vi "manual slider.vi"() -> ()   [LabVIEW 2020]
panel:
  out "Boolean 2":bool
  in  "Boolean":bool
  in  "stop":bool
  in  "VISA resource name":refnum<visa-resource-name>
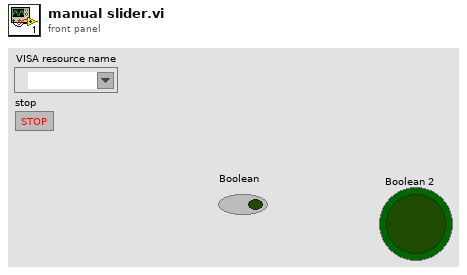
[diagram p1: front panel]
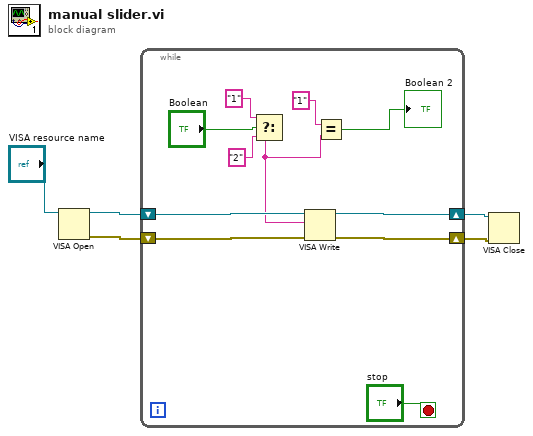
[diagram p0: block diagram]
diagram:
  n1 = VISA Open(VISA resource name="VISA resource name") -> (VISA resource name=w5:refnum<visa-resource-name>, error out=w4:errorcluster)  [unwired: 4 in]
  n2 = while {
    shift-right: [w14] -> w3
    shift-left: w5 -> [w16]
    shift-right: [w13] -> w2
    shift-left: w4 -> [w15]
    stop <- "stop" stop-if-true
    n3 = Select(t="1", s="Boolean", f="2") -> (s? t:f=w8:string)
    n4 = VISA Write(VISA resource name=w16, write buffer=w8, error in (no error)=w15) -> (VISA resource name out=w14:refnum<visa-resource-name>, error out=w13:errorcluster)  [unwired: 1 out]
    n5 = Equal?(x="1", y=w8) -> (x = y?=→"Boolean 2":bool)
  }
  n6 = VISA Close(VISA resource name=w3, error in (no error)=w2) -> ()  [unwired: 1 out]
